vi "Write Sondenmodell.Zustandsgrössen.vi"(8 "error in (no error)":errorcluster, 10 "Sondenmodell.Zustandsgrössen":T1, 11 "Sondenmodell in":refnum<class "Sondenmodell.lvclass">) -> (0 "error out":errorcluster, 3 "Sondenmodell out":refnum<class "Sondenmodell.lvclass">)   [LabVIEW 2016, in "Sondenmodell.lvclass"]
uses:
  Sondenmodell.lvclass
  Sondenmodell.lvclass/Sondenmodell.ctl
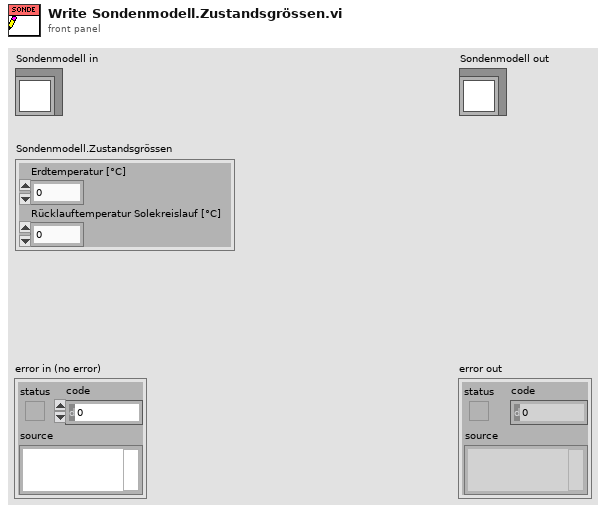
[diagram p1: front panel]
types:
  T1 = typedef "Sondenmodell.lvclass/Sondenmodell.Zustandsgrössen.ctl" = cluster{"Erdtemperatur [°C]":dbl, "Rücklauftemperatur Solekreislauf [°C]":dbl}
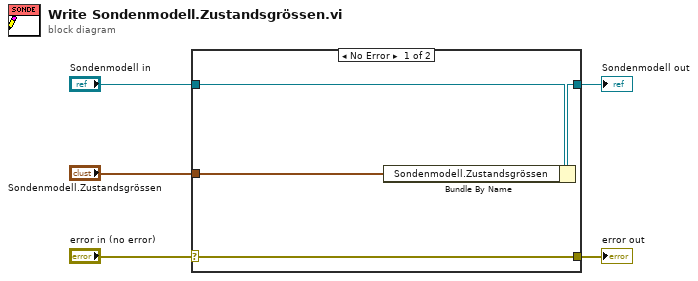
[diagram p0: block diagram]
diagram:
  n1 = case shown="No Error" "error in (no error)" {
    selector: "error in (no error)" -> [w9 w10]
    tunnel: [w9 w10] -> w4
    tunnel: [w7 w11] -> w2
    tunnel: "Sondenmodell in" -> [w8 w11]
    tunnel: "Sondenmodell.Zustandsgrössen" -> [w6 _]
    frame No Error {
      n2 = Bundle By Name(cluster=w8, "Sondenmodell.Zustandsgrössen"=w6) -> (w7:refnum<class "Sondenmodell.lvclass">)
    }
    frame Error {
    }
  }
  "error out" <- w4
  "Sondenmodell out" <- w2
